vi "AddTimeToArr.vi"(8 "Arr in":T1(array[cluster]), 11 "Cluster in":T2) -> (0 "Arr out":T1(array[cluster]), 3 "Cluster out":T2)   [LabVIEW 2017]
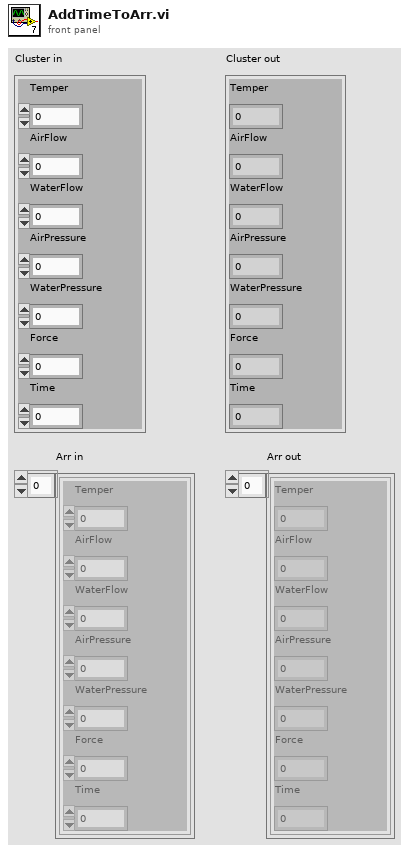
[diagram p1: front panel]
types:
  T1 = cluster{"Temper":dbl, "AirFlow":dbl, "WaterFlow":dbl, "AirPressure":dbl, "WaterPressure":dbl, "Force":dbl, "Time":dbl}[]
  T2 = cluster{"Temper":dbl, "AirFlow":dbl, "WaterFlow":dbl, "AirPressure":dbl, "WaterPressure":dbl, "Force":dbl, "Time":dbl}
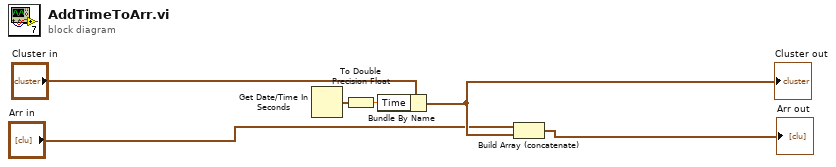
[diagram p0: block diagram]
diagram:
  n1 = Get Date/Time In Seconds() -> (seconds since 1Jan1904=w3:timestamp)
  n2 = To Double Precision Float(number=w3) -> (double precision float=w4:dbl)
  n3 = Bundle By Name(cluster="Cluster in", "Time"=w4) -> (w5:T2)
  "Cluster out" <- w5
  n4 = Build Array (concatenate)("Arr in", w5) -> (→"Arr out":T1)
